vi "Authentication Schemes Length.vi"(8 "Error In":errorcluster, 10 "Username":string, 11 "Session In":refnum<class "Session.lvclass">) -> (0 "Error Out":errorcluster, 2 "Length":i32, 3 "Sesssion Out":refnum<class "Session.lvclass">)   [LabVIEW 2021, in "Field_RnD_Services_LIBSSH2_Toolkit.lvlib" / "Session.lvclass"]
doc: "Gets the length in bytes (B) of the binary data returned for the supported authentication schemes for the remote SSH/SFTP server."
uses:
  Session.lvclass
  Field_RnD_Services_LIBSSH2_Toolkit.lvlib
  SSH/SSH.lvclass
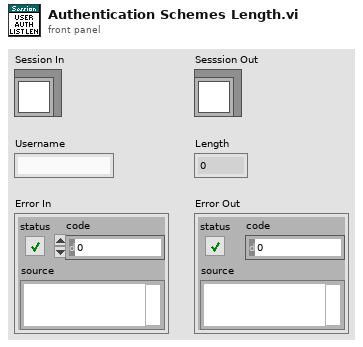
[diagram p1: front panel]
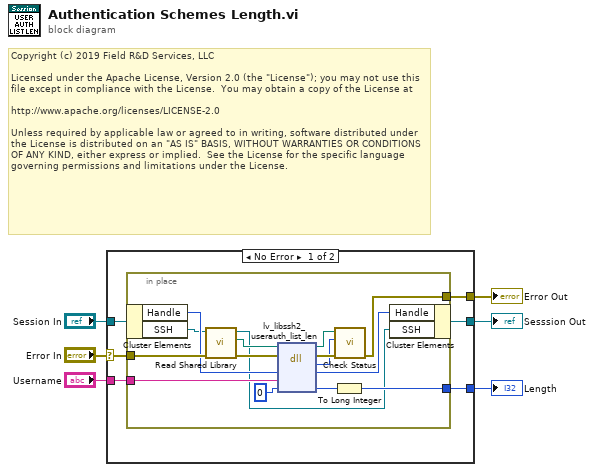
[diagram p0: block diagram]
diagram:
  # "Copyright (c) 2019 Field R&D Services, LLC\n\nLicensed under the Apache License, Version 2.0 (the \"License\"); you may not use this file except in compliance with the License.  You may obtain a copy of the License at\n\nhttp://www.apache.org/licenses/LICENSE-2.0\n\nUnless required by applicable law or agreed to in writing, software distributed under the License is distributed on an \"AS IS\" BASIS, WITHOUT WARRANTIES OR CONDITIONS OF ANY KIND, either express or implied.  See the License for the specific language governing permissions and limitations under the License."
  n1 = case shown="No Error" "Error In" {
    selector: "Error In" -> [w12 w29]
    tunnel: [w9 w29] -> w5
    tunnel: "Session In" -> [w11 w28]
    tunnel: [w10 w28] -> w3
    tunnel: [w8 _] -> w2
    tunnel: "Username" -> [w7 _]
    frame No Error {
      n2 = in-place {
        in-place-border: w12 -> [w24]
        in-place-border: [w23] -> w9
        in-place-border: [w22] -> w8
        in-place-border: w7 -> [w19]
        n3 = in-place-cluster #1(w11) -> ("Handle"=w18:u64, "SSH"=w15:refnum<class "SSH.lvclass">)
        n4 = call "Read Shared Library.vi"("Error In"=w24, "SSH In"=w15) -> ("Error Out"=w16:errorcluster, "libssh2lv Shared Library"=w14:path, "SSH Out"=w13:refnum<class "SSH.lvclass">)  [unwired: 7 in]
        n5 = dll-call lib="D:/Users/cfield/Code/Field R&D Services/SSH/LV-LIBSSH2/LabVIEW/trunk/src/Toolkit/Support/lv-libssh2.dll" fn="lv_libssh2_userauth_list_len"(path in=w14, error in=w16, "session"=w18, "username"=w19, "length"=u64 0) -> (path out=w26:path, error out=w27:errorcluster, "result"=w25:i32, "session"=w17:u64, "length"=w20:u64)  [unwired: 2 in]
        n6 = To Long Integer(number=w20) -> (32bit integer=w22:i32)
        n7 = call "Check Status.vi"("Error In"=w27, "Status"=w25, "libssh2lv Shared Library In"=w26) -> ("Error Out"=w23:errorcluster)  [unwired: 7 in, 1 out]
        n8 = in-place-cluster #1("Handle"=w17, "SSH"=w13) -> (w10:refnum<class "Session.lvclass">)
      }
    }
    frame Error {
    }
  }
  "Sesssion Out" <- w3
  "Error Out" <- w5
  "Length" <- w2
